vi "Untitled 2.vi"   [LabVIEW 2013]
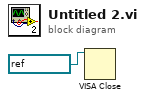
[diagram p0: block diagram]
diagram:
  n1 = VISA Close(VISA resource name=refnum<visa-resource-name> "COM3") -> ()  [unwired: 1 in, 1 out]
